vi "IMAQ Read Image File(Float32 Ex) With Vision Info.vi"(7 "File Path":path, 8 "error in (no error)":errorcluster, 11 "Image":T1) -> (0 "error out":errorcluster, 3 "Image (duplicate)":T1)   [LabVIEW 2020]
uses:
  <vilib>/vision/Image Controls.llb/IMAQ Image.ctl
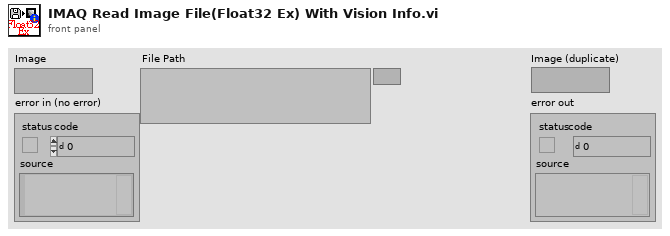
[diagram p1: front panel]
types:
  T1 = typedef "IMAQ Image.ctl" = refnum<image>
  T2 = typedef "Image Type" = u32
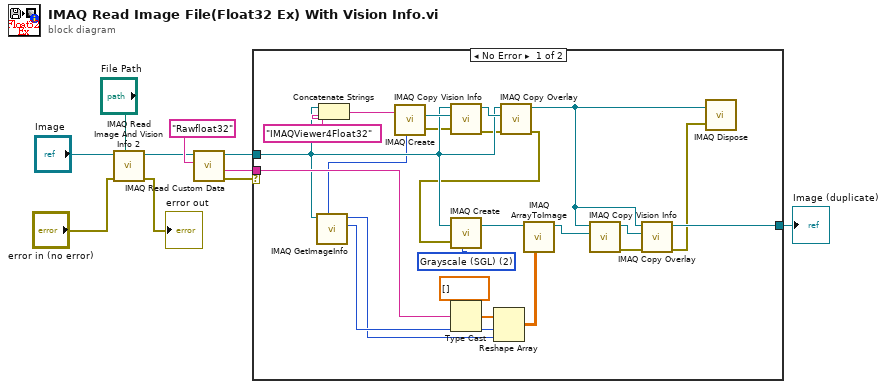
[diagram p0: block diagram]
diagram:
  n1 = call "IMAQ Read Image And Vision Info 2"("File Path"="File Path", "error in (no error)"="error in (no error)", "Image"="Image") -> ("error out"=→"error out":errorcluster, "Image Out"=w8:T1)  [unwired: 6 in, 1 out]
  n2 = call "IMAQ Read Custom Data"("Key"="Rawfloat32", "Image"=w8) -> ("error out"=w6:errorcluster, "Custom Data Out"=w9:string, "Image (duplicate)"=w7:T1)  [unwired: 7 in]
  n3 = case shown="No Error" w6 {
    tunnel: w9 -> [w33 _]
    tunnel: [w22 w34] -> w1
    tunnel: w7 -> [w17 w34]
    frame No Error {
      w30 = T2 2 items=["Grayscale (U8)", "Grayscale (I16)", "Grayscale (SGL)", "Complex (CSG)", "RGB (U32)", "HSL (U32)", "RGB (U64)", "Grayscale (U16)"] ("Image Type")
      n4 = call "IMAQ GetImageInfo"("Image"=w17) -> ("Y Resolution"=w28:i32, "X Resolution"=w27:i32, "Image Type"=w12:T2)  [unwired: 3 in, 5 out]
      n5 = Concatenate Strings(w17, "IMAQViewer4Float32" ("Image Name")) -> (w20:string)
      n6 = call "IMAQ Create"("Image Name"=w20, "Image Type"=w12) -> ("New Image"=w19:T1, "error out"=w16:errorcluster)  [unwired: 3 in]
      n7 = call "IMAQ Copy Vision Info"("error in (no error)"=w16, "Image Dst"=w19, "Image Src"=w17) -> ("error out"=w15:errorcluster, "Image Dst Out"=w18:T1)  [unwired: 6 in, 1 out]
      n8 = Type Cast(type=sgl[] [], x=w33) -> (*(type *) &x=w32:sgl[])
      n9 = Reshape Array(w32, w28, w27) -> (w31:sgl[][])
      n10 = call "IMAQ Copy Overlay"("error in (no error)"=w15, "Image Dst"=w18, "Image Src"=w17) -> ("error out"=w11:errorcluster, "Image Dst Out"=w13:T1)  [unwired: 7 in]
      n11 = call "IMAQ Create"("Image Name"=w17, "Image Type"=w30, "error in (no error)"=w11) -> ("New Image"=w29:T1)  [unwired: 2 in, 1 out]
      n12 = call "IMAQ ArrayToImage"("Image Pixels (Float)"=w31, "Image"=w29) -> ("Image Out"=w25:T1)  [unwired: 8 in, 1 out]
      n13 = call "IMAQ Copy Vision Info"("Image Dst"=w25, "Image Src"=w13) -> ("error out"=w24:errorcluster, "Image Dst Out"=w23:T1)  [unwired: 7 in, 1 out]
      n14 = call "IMAQ Copy Overlay"("error in (no error)"=w24, "Image Dst"=w23, "Image Src"=w13) -> ("error out"=w14:errorcluster, "Image Dst Out"=w22:T1)  [unwired: 7 in]
      n15 = call "IMAQ Dispose"("Image"=w13, "error in (no error)"=w14) -> ()  [unwired: 4 in, 1 out]
    }
    frame Error {
    }
  }
  "Image (duplicate)" <- w1
